vi "StateToString.vi"(11 "State Type Numeric":u32) -> (3 "State Type String":string)   [LabVIEW 2016, in "M1M3SupportEUI_Views.lvlib"]
uses:
  M1M3SupportEUI_Views.lvlib
  Typedefs/StateTypes.ctl
  Typedefs/M1M3SupportEUI_TypeDefs.lvlib
panel:
  out "State Types":T1 items=["Offline State"=0, "Fault State"=4294967295, "Standby State"=16777216, "Disabled State"=33554432, "Enabled State"=50331648, "Parked State"=50331649, "Raising State"=50331650, "Active State"=50331651, "Lowering State"=50331652, "Engineering State"=50397184, "Parked Engineering State"=50397185, "Raising Engineering State"=50397186, "Active Engineering State"=50397187, "Lowering Engineering State"=50397188]
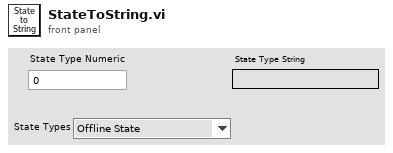
[diagram p1: front panel]
types:
  T1 = typedef "M1M3SupportEUI_TypeDefs.lvlib/StateTypes.ctl" = u32
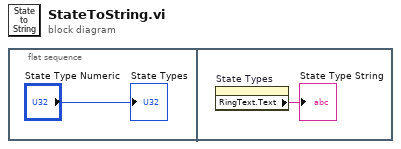
[diagram p0: block diagram]
diagram:
  n1 = flat-sequence {
    frame #0 {
      "State Types" <- "State Type Numeric"
    }
    frame #1 {
      n2 = property on="State Types" class="Ring (strict)"() -> ("RingText.Text"=→"State Type String":string)  [unwired: 2 in, 2 out]
    }
  }
